vi "CoreCMDs.vi"(8 "error in (no error)":errorcluster, 11 "BattPack in":refnum<class "Battery Pack.lvclass">) -> (0 "error out":errorcluster)   [LabVIEW 2021, in "Battery Pack.lvclass"]
uses:
  Battery Pack.lvclass
  C:/Program Files (x86)/National Instruments/LabVIEW 2021/user.lib/S2 Labs/Module Framework/Modules/Base/Module.lvclass
  C:/Program Files (x86)/National Instruments/LabVIEW 2021/user.lib/S2 Labs/Module Framework/Modules/Modbus/Modbus Slave Base/Modbus Slave Base.lvclass
  <userlib>/S2 Labs/Module Framework/Modules/Base/Module.lvclass/Module.ctl
  <userlib>/S2 Labs/Module Framework/Modules/Modbus/Modbus Slave Base/Modbus Slave Base.lvclass/Modbus Slave Base.ctl
  8f1a046c-3435-4d89-b670-d6766787dd10.vi
  f0c36d48-d948-4602-a448-2a739c09267b.vi
  <userlib>/S2 Labs/Module Framework/Modules/Modbus/Modbus Slave Base/Read MB Ref.vi
  1119e8ad-7c01-4eec-8c8e-616206ad473d.vi
  <userlib>/S2 Labs/Module Framework/Modules/Base/Read Name.vi
  <userlib>/S2 Labs/Error Reporting/ER Global.vi
  <userlib>/S2 Labs/Error Reporting/Error Reporting Class/subVIs/Report Error.vi
  <vilib>/Utility/error.llb/Error Cluster From Error Code.vi
  <userlib>/S2 Labs/Modbus Toolkit/Slave/S2L Modbus Slave.lvclass
  <userlib>/S2 Labs/Queued State Machine/QSM.lvclass
  <userlib>/S2 Labs/Module Framework/Modules/Base/Module.lvclass
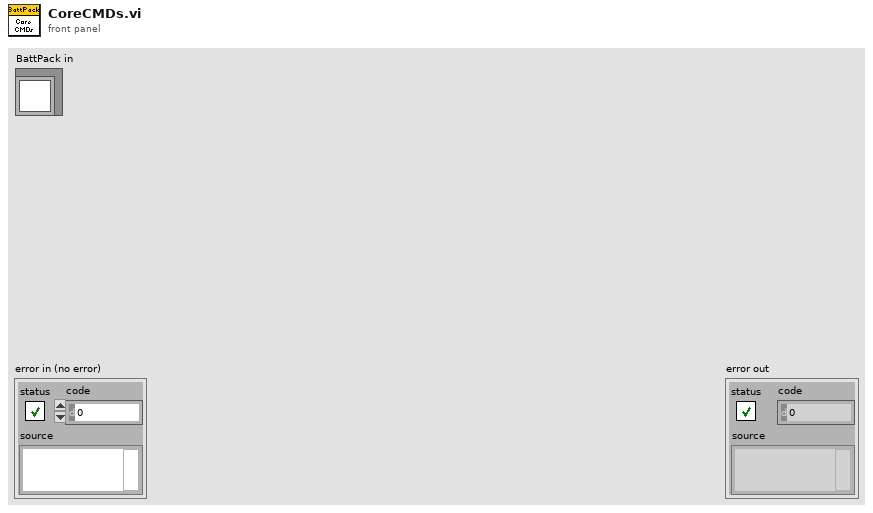
[diagram p1: front panel]
types:
  T1 = typedef "QSM.lvclass/Queue Message.ctl" = cluster{"State":T2, "Command":string, "Parameter":variant}
  T2 = typedef "QSM.lvclass/States.ctl" = enum16{"Waiting", "Init", "ExecCMD", "Read Config", "Write Config", "Launch", "Connect", "Recovery", "Clean Up", "Exit"}
  T3 = typedef "QSM.lvclass/CallbackNotifierRef.ctl" = refnum<class "Callback Notifier.lvclass">
  T4 = cluster{"Callback Requested?":bool, "Callback Notifier out":T3}
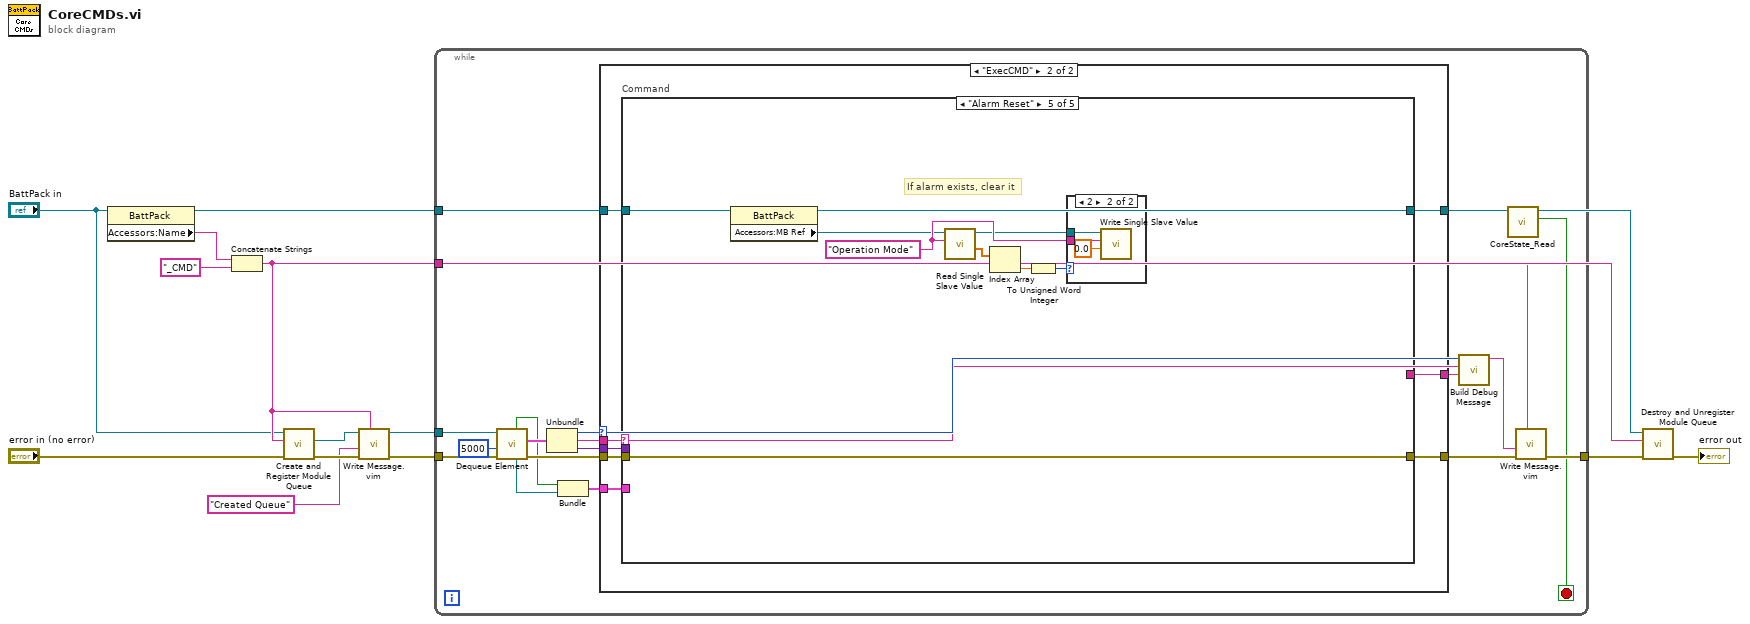
[diagram p0: block diagram]
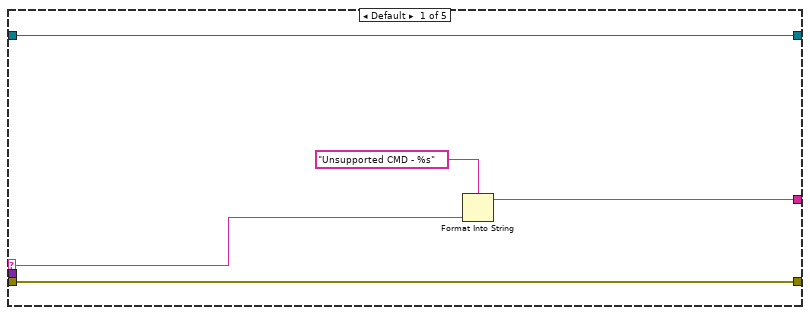
[diagram p3: hidden frame]
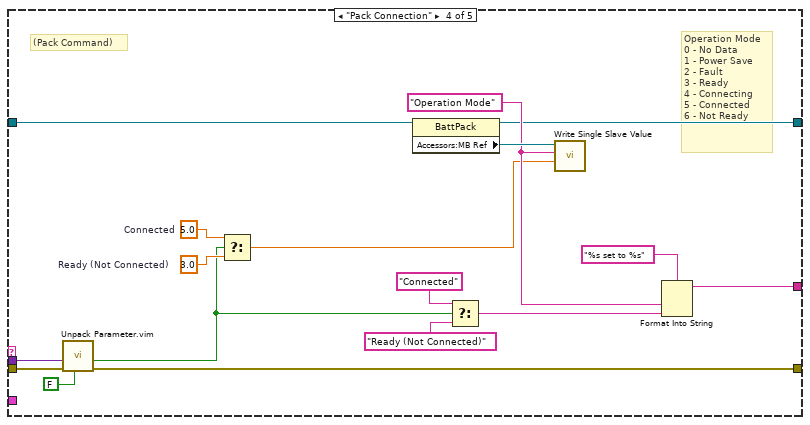
[diagram p6: hidden frame]
diagram:
  n1 = property class="BattPack"(reference="BattPack in") -> (reference out=w11:refnum<class "Battery Pack.lvclass">, "Accessors:Name"=w6:string)  [unwired: 1 in, 1 out]
  n2 = Concatenate Strings(w6, "_CMD") -> (w12:string)
  n3 = call <userlib>:"Create and Register Module Queue.vi"("error in (no error)"="error in (no error)", "Name"=w12, "Module in"="BattPack in") -> ("error out"=w9:errorcluster, "Queue Reference"=w4:refnum<class "QSM.lvclass">)  [unwired: 6 in, 1 out]
  n4 = call "Write Message.vim"("Message Tag"=w12, "error in (no error)"=w9, "Message (string)"="Created Queue") -> ("error out"=w8:errorcluster)  [unwired: 8 in]
  n5 = while {
    tunnel: w8 -> [w29]
    tunnel: w12 -> [w26]
    tunnel: w11 -> [w27]
    tunnel: [w28] -> w10
    tunnel: w4 -> [w13]
    stop <- w23 stop-if-true
    n6 = call <userlib>:"Dequeue Element.vi"("error in (no error)"=w29, "timeout in ms (-1)"=5000, "QSM in"=w13) -> ("error out"=w22:errorcluster, "Message"=w31:T1, "Callback Notifier out"=w15:T3, "Callback Requested?"=w16:bool)  [unwired: 3 in, 2 out]
    n7 = Unbundle(w31) -> ("State"=w20:T2, "Command"=w19:string, "Parameter"=w25:variant)
    n8 = Bundle("Callback Requested?"=w16, "Callback Notifier out"=w15) -> (w14:T4)  [unwired: 1 in]
    n9 = case shown="\"ExecCMD\"" w20 {
      tunnel: w27 -> [w33 w35]
      tunnel: [w33 w36] -> w24
      tunnel: w19 -> [_ w41]
      tunnel: w25 -> [_ w40]
      tunnel: w22 -> [w32 w39]
      tunnel: [w32 w38] -> w21
      tunnel: [_ w37] -> w18
      tunnel: w14 -> [_ w34]
      frame Default {
      }
      frame "ExecCMD" {
        n10 = case "Command" shown="\"Alarm Reset\"" w41 {
          selector: w41 -> [w44 _ _ _ _]
          tunnel: w40 -> [_ _ _ w67 _]
          tunnel: w39 -> [w46 w47 w49 w61 w68]
          tunnel: [w46 w47 w49 w60 w68] -> w38
          tunnel: [w42 _ _ w54 _] -> w37
          tunnel: [w45 w48 w50 w51 w69] -> w36
          tunnel: w35 -> [w45 w48 w50 w63 w70]
          tunnel: w34 -> [_ _ _ _ _]
          frame Default {
            n11 = Format Into String(format string="Unsupported CMD - %s" ("<JSON>"), w44) -> (resulting string=w42:string)  [unwired: 2 in, 1 out]
          }
          frame "System alarm reset CMD" {
          }
          frame "System connection CMD" {
          }
          frame "Pack Connection" {
            w64 = 3.0  # Ready (Not Connected)
            w65 = 5.0  # Connected
            w53 = "Operation Mode"
            # "(Pack Command)"
            # "Operation Mode\n0 - No Data\n1 - Power Save\n2 - Fault\n3 - Ready\n4 - Connecting\n5 - Connected\n6 - Not Ready"
            n12 = call "Unpack Parameter.vim"("Parameter type (string)"=FALSE, "error in"=w61, "Parameter Variant"=w67) -> ("error out"=w60:errorcluster, "Parameter"=w59:bool)  [unwired: 7 in]
            n13 = Select(t=w65, s=w59, f=w64) -> (s? t:f=w52:dbl)
            n14 = property class="BattPack"(reference=w63) -> (reference out=w51:refnum<class "Battery Pack.lvclass">, "Accessors:MB Ref"=w62:refnum<class "S2L Modbus Slave.lvclass">)  [unwired: 1 in, 1 out]
            n15 = Select(t="Connected", s=w59, f="Ready (Not Connected)") -> (s? t:f=w55:string)
            n16 = call-dynamic "Write Single Slave Value.vi"("Value"=w52, "Label"=w53, "S2L Modbus Slave in"=w62) -> ()  [unwired: 7 in, 2 out]
            n17 = Format Into String(format string="%s set to %s", w53, w55) -> (resulting string=w54:string)  [unwired: 2 in, 1 out]
          }
          frame "Alarm Reset" {
            w73 = "Operation Mode"
            # "If alarm exists, clear it"
            n18 = property class="BattPack"(reference=w70) -> (reference out=w69:refnum<class "Battery Pack.lvclass">, "Accessors:MB Ref"=w71:refnum<class "S2L Modbus Slave.lvclass">)  [unwired: 1 in, 1 out]
            n19 = call-dynamic "Read Single Slave Value.vi"("Label"=w73, "S2L Modbus Slave in"=w71) -> ("Value (s)"=w74:dbl[], "S2L Modbus Slave out"=w72:refnum<class "S2L Modbus Slave.lvclass">)  [unwired: 4 in, 4 out]
            n20 = Index Array(array=w74) -> (element=w75:dbl)  [unwired: 1 in]
            n21 = To Unsigned Word Integer(number=w75) -> (unsigned 16bit integer=w76:u16)
            n22 = case shown="2" w76 {
              tunnel: w72 -> [_ w79]
              tunnel: w73 -> [_ w78]
              frame Default {
              }
              frame 2 {
                n23 = call-dynamic "Write Single Slave Value.vi"("Value"=0.0, "Label"=w78, "S2L Modbus Slave in"=w79) -> ()  [unwired: 7 in, 2 out]
              }
            }
          }
        }
      }
    }
    n24 = call <userlib>:"Build Debug Message.vi"("Debug Message"=w18, "Command"=w19, "State"=w20) -> ("Built Message"=w17:string)  [unwired: 8 in]
    n25 = call-dynamic "CoreState_Read.vi"("Module in"=w24) -> ("Stopped?"=w23:bool)  [unwired: 8 in, 2 out]
    n26 = call "Write Message.vim"("Message Tag"=w26, "error in (no error)"=w21, "Message (string)"=w17) -> ("error out"=w28:errorcluster)  [unwired: 8 in]
  }
  n27 = call <userlib>:"Destroy and Unregister Module Queue.vi"("error in (no error)"=w10, "Name"=w12, "Module in"=w11) -> ("error out"=→"error out":errorcluster)  [unwired: 7 in, 1 out]
